vi "[FPGA] IP Builder - Float Transfer Function.vi"(5 "TF Order":i32=2, 7 "Den":sgl[](array[numeric])=[0.982758, -1.98194, 1.0, 0.0, 0.0, 0.0, 0.0, 0.0, 0.0], 8 "Num":sgl[](array[numeric])=[-0.00254, 0.000408, 0.00295, 0.0, 0.0, 0.0, 0.0, 0.0, 0.0], 9 "State In":sgl[](array[numeric])=[0.0, 0.0, 0.0, 0.0, 0.0, 0.0, 0.0, 0.0, 0.0], 10 "Input":sgl) -> (2 "State Out":sgl[](array[numeric]), 3 "Output":sgl)   [LabVIEW 2017]
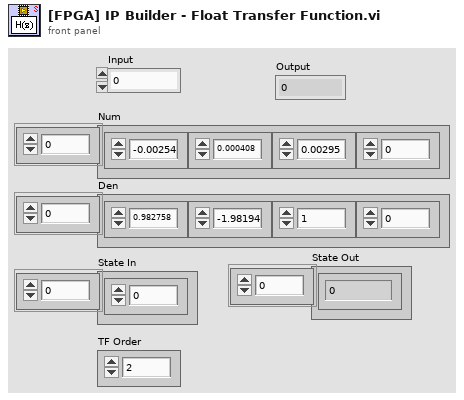
[diagram p1: front panel]
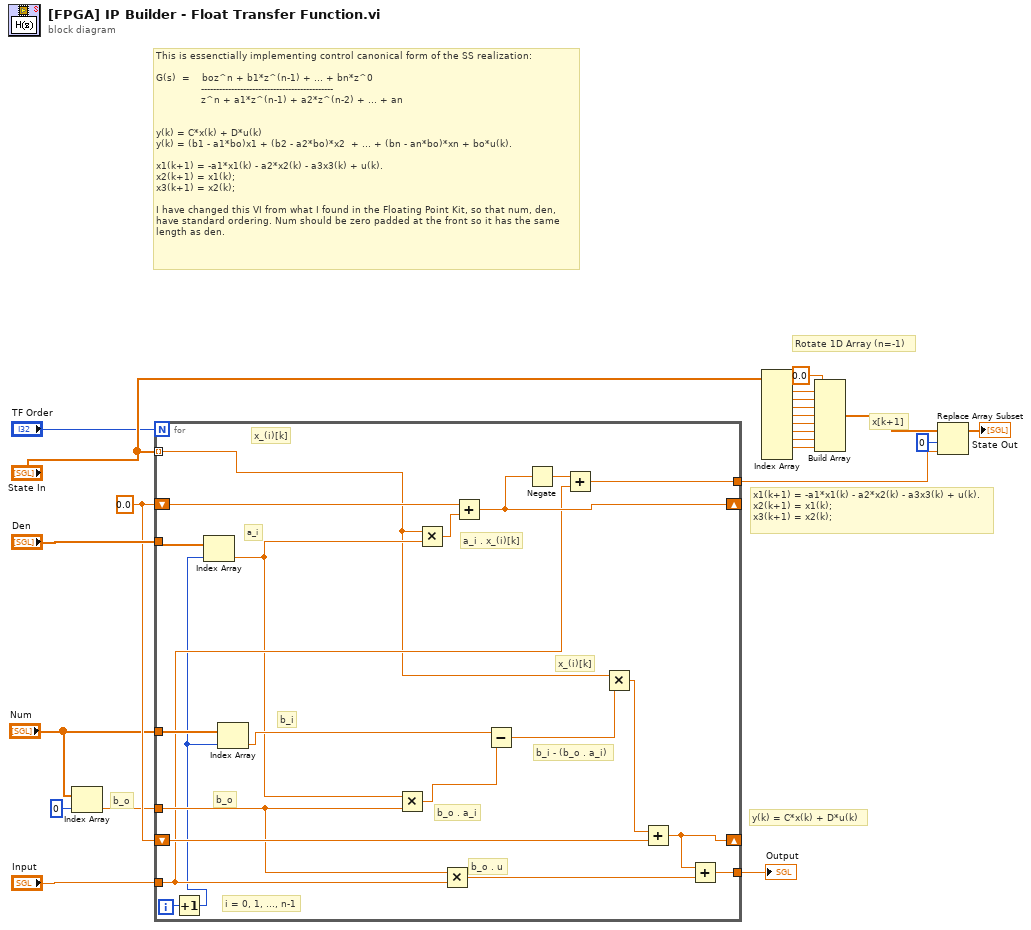
[diagram p0: block diagram]
diagram:
  w16 = sgl 0.0 ("element")
  # "x1(k+1) = -a1*x1(k) - a2*x2(k) - a3x3(k) + u(k).\nx2(k+1) = x1(k);\nx3(k+1) = x2(k);"
  # "y(k) = C*x(k) + D*u(k)"
  # "This is essenctially implementing control canonical form of the SS realization:\n\nG(s)  =    boz^n + b1*z^(n-1) + ... + bn*z^0\n               --------------------------------------------\n               z^n + a1*z^(n-1) + a2*z^(n-2) + ... + an\n\n\ny(k) = C*x(k) + D*u(k)\ny(k) = (b1 - a1*bo)x1 + (b2 - a2*bo)*x2  + ... + (bn - an*bo)*xn + bo*u(k).\n\nx1(k+1) = -a1*x1(k) - a2*x2(k) - a3x3(k) + u(k).\nx2(k+1) = x1(k);\nx3(k+1) = x2(k);\n\nI have changed this VI from what I found in the Floating Point Kit, so that num, den, have standard ordering. Num should be zero padded at the front so it has the same length as den."
  # "b_o"
  # "Rotate 1D Array (n=-1)"
  # "x[k+1]"
  n1 = Index Array(array="Num", index=0) -> (element=w14:sgl)
  n2 = for {
    N: "TF Order" -> [_]
    tunnel: "Den" -> [w27]
    shift-right: [w33] -> _
    shift-left: w16 -> [w43]
    tunnel: "Num" -> [w32]
    shift-right: [w39] -> _
    shift-left: w16 -> [w42]
    tunnel: "Input" -> [w31]
    tunnel: [w37] -> w20
    tunnel: [w34] -> w18
    tunnel: w14 -> [w35]
    tunnel: "State In" -> [w25] mode=indexing
    i -> [w30]
    # "x_(i)[k]"
    # "b_o . u"
    # "b_o"
    # "i = 0, 1, ..., n-1"
    # "x_(i)[k]"
    # "b_i - (b_o . a_i)"
    # "b_o . a_i"
    # "b_i"
    # "a_i . x_(i)[k]"
    # "a_i"
    n3 = Increment(x=w30) -> (x+1=w26:i32)
    n4 = Index Array(array=w27, index=w26) -> (element=w28:sgl)
    n5 = Index Array(array=w32, index=w26) -> (element=w29:sgl)
    n6 = Multiply(x=w28, y=w35) -> (x*y=w40:sgl)
    n7 = Multiply(x=w25, y=w28) -> (x*y=w41:sgl)
    n8 = Multiply(x=w35, y=w31) -> (x*y=w38:sgl)
    n9 = Add(x=w43, y=w41) -> (x+y=w33:sgl)
    n10 = Subtract(x=w29, y=w40) -> (x-y=w24:sgl)
    n11 = Negate(x=w33) -> (-x=w36:sgl)
    n12 = Add(x=w36, y=w31) -> (x+y=w34:sgl)
    n13 = Multiply(x=w25, y=w24) -> (x*y=w23:sgl)
    n14 = Add(x=w23, y=w42) -> (x+y=w39:sgl)
    n15 = Add(x=w39, y=w38) -> (x+y=w37:sgl)
  }
  "Output" <- w20
  n16 = Index Array(array="State In") -> (element #1=w3:sgl, element #2=w4:sgl, element #3=w5:sgl, element #4=w6:sgl, element #5=w7:sgl, element #6=w8:sgl, element #7=w9:sgl, element #8=w10:sgl)  [unwired: 9 in, 1 out]
  n17 = Build Array(sgl 0.0 ("element"), w3, w4, w5, w6, w7, w8, w9, w10) -> (w19:sgl[])
  n18 = Replace Array Subset(array=w19, new element=w18, index=0) -> (→"State Out":sgl[])
